vi "Queue MultiPakect-13.vi"(8 "no error":errorcluster, 10 "VISA resource name - IN":refnum<visa-resource-name>="COM4", 11 "EndSession":bool=TRUE) -> (0 "error out":errorcluster={"status"=FALSE, "code"=1073676294, "source"="VISA Read in SerialCOM.vi->Queue MultiPakect-13.vi->getvideo.vi->Focus Routine.vi->Focus Routine.vi.ProxyCaller"}, 1 "success?":bool=TRUE, 2 "ImageData":u8[](array[numeric]) format="%x", 5 "RecvBuff":string, 6 "Done":bool=TRUE, 9 "VISA resource name - OUT":refnum<visa-resource-name>="COM4")   [LabVIEW 2014]
doc: "Demonstrates general use of Obtain Queue, queues and the effects different settings have on queue behavior. It uses a queue to pass data between an Enqueue loop (producing data) and a Dequeue loop (consuming data). If both loops run at the same speed, the queue does not fill up.\n\nWhen the Enqueue loop runs fast and the Dequeue loop runs slow, the queue quickly fills up and the Enqueue loop must wait for the Dequeue loop to remove elements. If the Enqueue loop runs slow and the Dequeue loop runs fast, the queue is quickly emptied and the Dequeue loop must wait for the Enqueue loop to insert elements."
panel:
  out "SendEndSession":bool
  out "max":u32
  out "Raw Data":u8[](array[numeric]) format="%x"
  out "Num_images":dbl=2.0
  out "readtime 2":u32=395
  out "RecvBuff 2":string
  out "ACK 2":bool=TRUE
  out "ACK":bool
  out "#Ends":u32
  out "source":string="VISA Read in SerialCOM.vi->Queue MultiPakect-13.vi->getvideo.vi->Focus Routine.vi->Focus Routine.vi.ProxyCaller"
  out "Pakect":u8[](array[numeric])=[152, 180, 0, 0, 18, 18, 18, 18, 19, 18, 19, 18, 18, 19, 18, 19, 18, 18, 18, 18, 18, 19, 18, 18, 18, 18, 18, 18, 18, 18, 18, 18, 18, 18, 19, 18, 19, 18, 18, 18, 18, 18, 19, 18, 18, 18, 18, 18, 18, 18, 18, 18, 19, 19, 18, 18, 18, 18, 19, 19, 18, 19, 18, 18, 18, 18, 18, 18, 18, 18, 18, 18, 19, 18, 19, 18, 19, 18, 19, 18, 18, 18, 18, 19, 18, 19, 18, 18, 18, 19, 19, 18, 18, 18, 18, 18, 18, 18, 18, 18, 18, 19, 18, 18, 18, 18, 18, 18, 19, 18, 18, 18, 19, 18, 18, 18, 19, 19, 18, 18, 18, 18, 19, 19, 18, 18, 18, 19, 19, 18, 18, 18, 18, 19, 18, 18, 18, 18, 18, 18, 18, 18, 18, 19, 18, 18, 18, 19, 18, 18, 18, 18, 244, 43]
  out "End paks":bool=TRUE
  out "Index":u32=200346
  out "#Pakects":u32=783
  out "# in queue":i32
  out "readtime":u32=395
  out "DeEnque Loop":i32=879
  out "StartTime":u32=22222026
  out "Bytes At Port Loop":i32=1757
  out "Bytes at Port":u32
  out "Enque Loop":i32=391
  out "Bytes Read":u32=200346
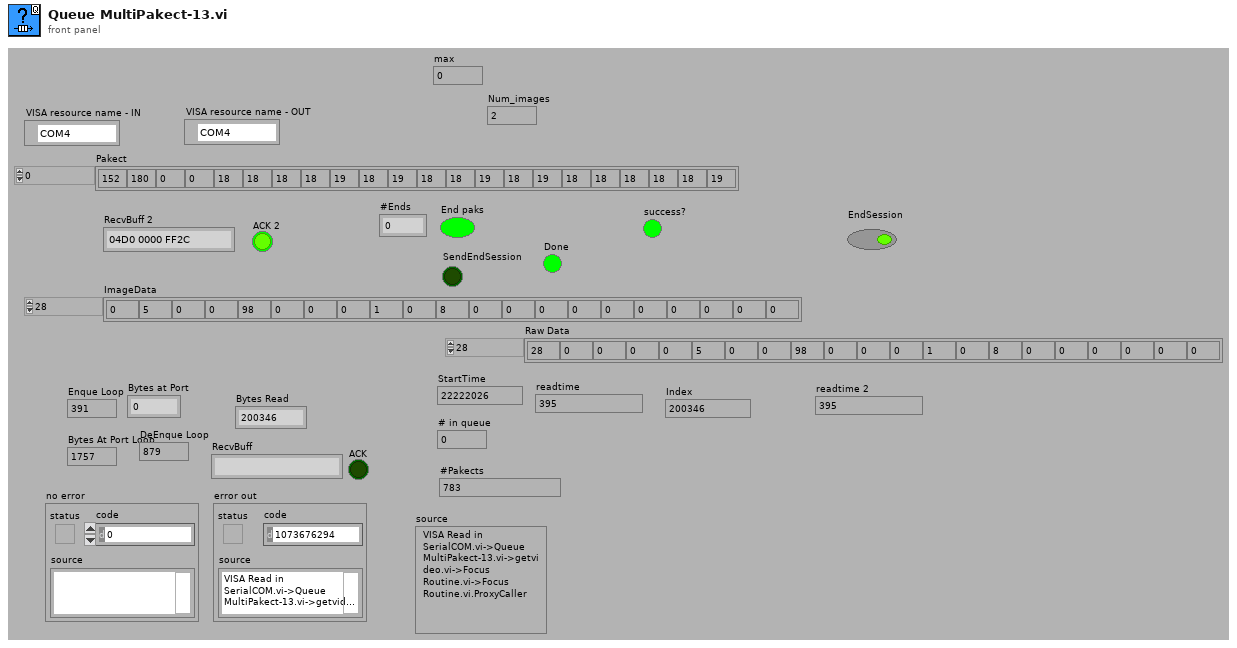
[diagram p1: front panel]
types:
  T1 = enum16{"OpenPort", "Initial Serial Port", "Write", "ByteRead", "Read", "ClearBuff", "Close"}
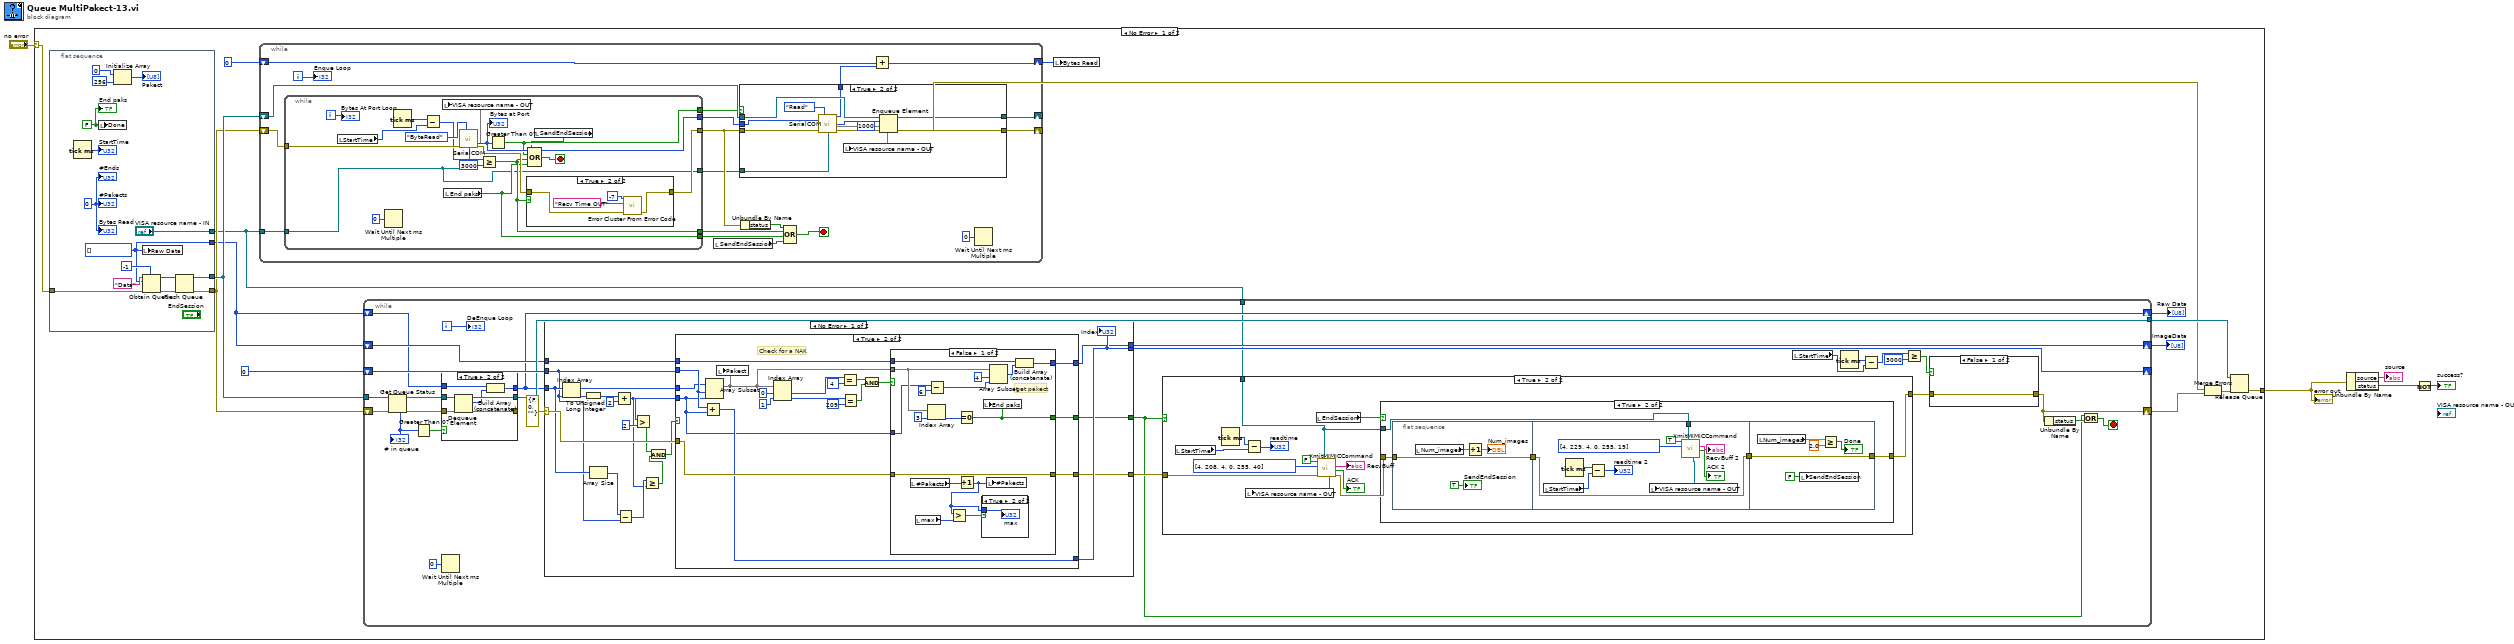
[diagram p0: block diagram]
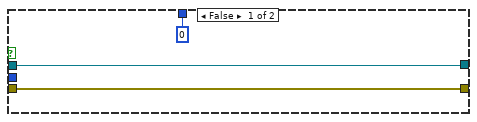
[diagram p3: hidden frame]
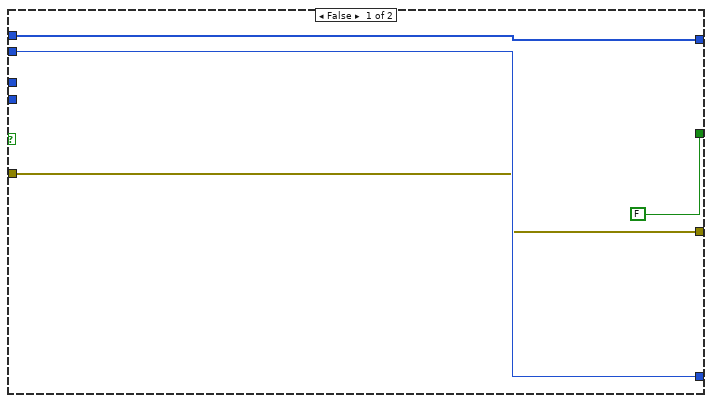
[diagram p4: hidden frame]
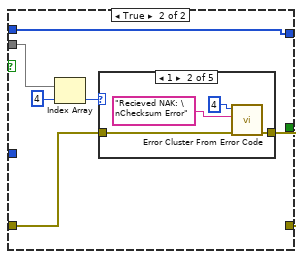
[diagram p6: hidden frame]
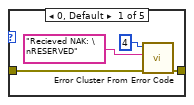
[diagram p7: hidden frame]
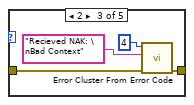
[diagram p8: hidden frame]
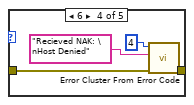
[diagram p9: hidden frame]
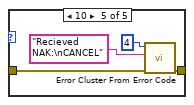
[diagram p10: hidden frame]
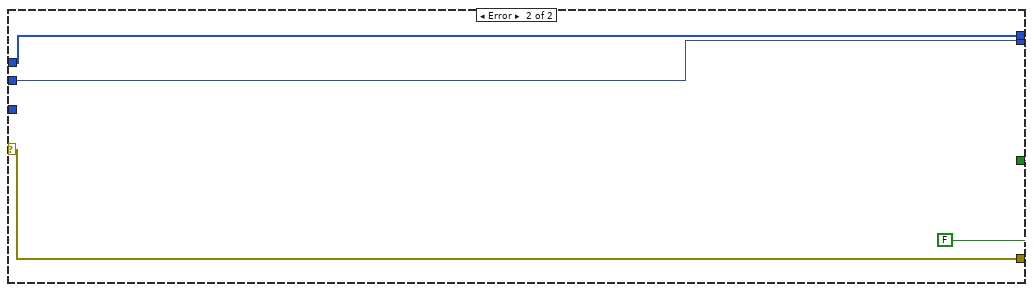
[diagram p11: hidden frame]
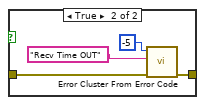
[diagram p12: hidden frame]
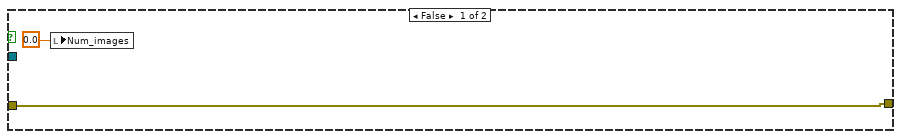
[diagram p15: hidden frame]
diagram:
  n1 = case shown="No Error" "no error" {
    selector: "no error" -> [w11 w264]
    tunnel: [w10 w264] -> w2
    frame No Error {
      n2 = flat-sequence {
        tunnel: [w31] -> w17
        tunnel: [w29] -> w9
        tunnel: [w28] -> w7
        tunnel: w11 -> [w23]
        tunnel: ["VISA resource name - IN"] -> w6
        frame #0 {
          w22 = u32 0 ("Bytes Read")
          w24 = FALSE ("full")
          w28 = u8[] []
          n3 = Tick Count (ms)() -> (millisecond timer value=→"StartTime":u32)
          n4 = local write "Done"(w24) -> ()
          n5 = Initialize Array(u8 0 ("element"), 256 ("dimension size")) -> (→"Pakect":u8[])
          n6 = local write "Raw Data"(w28) -> ()
          n7 = Obtain Queue(max queue size (-1, unlimited)=-1, name (unnamed)="Data", element data type=w28, error in (no error)=w23) -> (queue out=w32:refnum<queue>, error out=w30:errorcluster)  [unwired: 1 in, 1 out]
          n8 = Flush Queue(queue=w32, error in (no error)=w30) -> (queue out=w31:refnum<queue>, error out=w29:errorcluster)  [unwired: 1 out]
          "Bytes Read" <- w22
          "#Pakects" <- w22
          "End paks" <- w24
          "#Ends" <- w22
        }
      }
      n9 = while {
        shift-right: [w51] -> w20
        shift-left: u32 0 ("Bytes Read") -> [w53]
        shift-right: [w49] -> w14
        shift-left: w9 -> [w50]
        shift-right: [w43] -> _
        shift-left: w17 -> [w54]
        tunnel: w6 -> [w39]
        i -> [w47]
        stop <- w48 stop-if-true
        n10 = while {
          tunnel: [w62] -> w45
          tunnel: [w64] -> w52
          tunnel: w50 -> [w71]
          tunnel: [w61] -> w46
          tunnel: [w59] -> w44
          tunnel: [w60] -> w41
          tunnel: w39 -> [w58]
          tunnel: [w58] -> w38
          i -> [w70]
          stop <- w65 stop-if-true
          n11 = local read "StartTime"() -> (w68:u32)
          n12 = Wait Until Next ms Multiple(millisecond multiple=u32 0 ("milliseconds to wait")) -> ()  [unwired: 1 out]
          n13 = Tick Count (ms)() -> (millisecond timer value=w69:u32)
          n14 = Subtract(x=w69, y=w68) -> (x-y=w67:u32)
          n15 = local read "End paks"() -> (w59:bool)
          n16 = call "SerialCOM.vi"("Function"=T1."ByteRead", "error in (no error)"=w71, "VISA_IN"=w58) -> ("Bytes at Port"=w64:u32, 14:w57, "error out"=w63:errorcluster)  [unwired: 6 in, 4 out]
          "Bytes at Port" <- w64
          n17 = local write "VISA resource name - OUT"(w57) -> ()
          n18 = Greater Or Equal?(x=w67, y=u32 3000) -> (x >= y?=w60:bool)
          n19 = Greater Than 0?(x=w64) -> (x > 0?=w61:bool)
          n20 = case shown="True" w60 {
            tunnel: w63 -> [w73 w77]
            tunnel: [w73 w76] -> w62
            frame False {
            }
            frame True {
              n21 = call <vilib>:"Error Cluster From Error Code.vi"("error in (no error)"=w77, "error message (\"\")"="Recv Time OUT" ("error message (\"\")"), "error code (0)"=-7) -> ("error out"=w76:errorcluster)  [unwired: 6 in]
            }
          }
          n22 = local read "SendEndSession"() -> (w55:bool)
          n23 = Compound Arithmetic op=OR(w55, w61, w60, w59) -> (w65:bool)
          "Bytes At Port Loop" <- w70
        }
        n24 = local read "SendEndSession"() -> (w37:bool)
        n25 = case shown="True" w46 {
          tunnel: w45 -> [w80 w89]
          tunnel: w52 -> [_ w87]
          tunnel: w54 -> [w79 w91]
          tunnel: [w80 w85] -> w49
          tunnel: [w79 w86] -> w43
          tunnel: [u32 0 ("return count") w88] -> w42
          tunnel: w38 -> [_ w83]
          frame False {
          }
          frame True {
            n26 = call "SerialCOM.vi"("Function"=T1."Read", "byte count"=w87, "error in (no error)"=w89, "VISA_IN"=w83) -> ("return count"=w88:u32, "array Out"=w84:u8[], 14:w82, "error out"=w90:errorcluster)  [unwired: 5 in, 3 out]
            n27 = local write "VISA resource name - OUT"(w82) -> ()
            n28 = Enqueue Element(queue=w91, element=w84, timeout in ms (-1)=1000, error in (no error)=w90) -> (queue out=w86:refnum<queue>, error out=w85:errorcluster)  [unwired: 1 out]
          }
        }
        n29 = Unbundle By Name(w45) -> ("status"=w40:bool)
        n30 = Compound Arithmetic op=OR(w40, w41, w44, w37) -> (w48:bool)
        n31 = Add(x=w53, y=w42) -> (x+y=w51:u32)
        n32 = Wait Until Next ms Multiple(millisecond multiple=u32 0 ("milliseconds to wait")) -> ()  [unwired: 1 out]
        "Enque Loop" <- w47
      }
      n33 = while {
        tunnel: w17 -> [w119]
        tunnel: [w114] -> w18
        shift-right: [w106] -> w13
        shift-left: w9 -> [w120]
        shift-right: [w113] -> _
        shift-left: u32 0 ("#Pakects") -> [w117]
        shift-right: [w104] -> w12
        shift-left: w7 -> [w105]
        shift-right: [w97] -> w8
        shift-left: w7 -> [w96]
        tunnel: w6 -> [w94]
        i -> [w118]
        stop <- w101 stop-if-true
        n34 = Get Queue Status(queue=w119, error in (no error)=w120) -> (queue out=w115:refnum<queue>, error out=w116:errorcluster, # elements in queue=w98:i32)  [unwired: 1 in, 5 out]
        "# in queue" <- w98
        n35 = Greater Than 0?(x=w98) -> (x > 0?=w99:bool)
        n36 = Wait Until Next ms Multiple(millisecond multiple=u32 0 ("milliseconds to wait")) -> ()  [unwired: 1 out]
        n37 = case shown="True" w99 {
          tunnel: w116 -> [w215 w218]
          tunnel: [w215 w217] -> _
          tunnel: w115 -> [w216 w223]
          tunnel: [w216 w222] -> w114
          tunnel: w96 -> [w214 w221]
          tunnel: [w214 w219] -> w97
          frame False {
          }
          frame True {
            n38 = Dequeue Element(queue=w223, error in (no error)=w218) -> (queue out=w222:refnum<queue>, element=w220:u8[], error out=w217:errorcluster)  [unwired: 2 out]
            n39 = Build Array (concatenate)(w221, w220) -> (w219:u8[])
          }
        }
        n40 = case shown="No Error" errorcluster {"status"=FALSE, "code"=0, "source"=""} ("error IO") {
          selector: errorcluster {"status"=FALSE, "code"=0, "source"=""} ("error IO") -> [w129 w208]
          tunnel: w117 -> [w121 w206]
          tunnel: [w135 w206] -> w113
          tunnel: [w134 w208] -> w112
          tunnel: w105 -> [w132 w207]
          tunnel: [w131 w207] -> w104
          tunnel: w97 -> [w128 _]
          tunnel: [w130 FALSE] -> w102
          frame No Error {
            n41 = Index Array(array=w128, index=w121) -> (element=w136:u8)
            n42 = To Unsigned Long Integer(number=w136) -> (unsigned 32bit integer=w137:u32)
            n43 = Array Size(array=w128) -> (size(s)=w127:i32)
            n44 = Add(x=w137, y=u32 2) -> (x+y=w122:u32)
            n45 = Subtract(x=w127, y=w121) -> (x-y=w123:u32)
            n46 = Greater?(x=w122, y=u32 2) -> (0:w126:bool)
            n47 = Greater Or Equal?(x=w123, y=w122) -> (x >= y?=w125:bool)
            n48 = And(x=w126, y=w125) -> (x .and. y?=w124:bool)
            n49 = case shown="True" w124 {
              tunnel: [w139 w155] -> w131
              tunnel: w121 -> [w141 w153]
              tunnel: w129 -> [w140 w152]
              tunnel: [w141 w148] -> w135
              tunnel: [w140 w147] -> w134
              tunnel: w128 -> [_ w146]
              tunnel: [FALSE w145] -> w130
              tunnel: w122 -> [_ w144]
              tunnel: w132 -> [w139 w143]
              frame False {
              }
              frame True {
                # "Check for a NAK"
                n50 = Add(x=w153, y=w144) -> (x+y=w148:u32)
                n51 = Array Subset(array=w146, index=w153, length=w144) -> (w149:u8[])
                n52 = local write "Pakect"(w149) -> ()
                n53 = Index Array(array=w149, index #1=0 ("index"), index #2=1 ("index")) -> (element #1=w161:u8, element #2=w150:u8)
                n54 = Equal?(x=w161, y=u8 4) -> (x = y?=w157:bool)
                n55 = Equal?(x=w150, y=u8 209) -> (x = y?=w158:bool)
                n56 = Compound Arithmetic op=AND(w157, w158) -> (w154:bool)
                n57 = case shown="False" w154 {
                  tunnel: [w168 w179] -> w155
                  tunnel: w149 -> [w172 w182]
                  tunnel: w144 -> [w171 _]
                  tunnel: w152 -> [w174 w184]
                  tunnel: [w174 w180] -> w147
                  tunnel: [w166 _] -> w145
                  tunnel: w143 -> [w167 w179]
                  frame False {
                    # "get pakect"
                    n58 = local read "#Pakects"() -> (w165:u32)
                    n59 = local read "max"() -> (w162:u32)
                    n60 = Subtract(x=w171, y=u32 6) -> (x-y=w175:u32)
                    n61 = Index Array(array=w172, index=3) -> (element=w170:u8)
                    n62 = Equal To 0?(x=w170) -> (x = 0?=w166:bool)
                    n63 = Increment(x=w165) -> (x+1=w163:u32)
                    n64 = Greater?(x=w163, y=w162) -> (0:w164:bool)
                    n65 = case shown="True" w164 {
                      tunnel: w163 -> [_ w178]
                      frame False {
                      }
                      frame True {
                        "max" <- w178
                      }
                    }
                    n66 = local write "End paks"(w166) -> ()
                    n67 = local write "#Pakects"(w163) -> ()
                    n68 = Array Subset(array=w172, index=4, length=w175) -> (w169:u8[])
                    n69 = Build Array (concatenate)(w167, w169) -> (w168:u8[])
                  }
                  frame True {
                    n70 = Index Array(array=w182, index=4) -> (element=w181:u8)
                    n71 = case shown="1" w181 {
                      tunnel: w184 -> [w188 w192 w196 w200 w204]
                      tunnel: [w187 w191 w195 w199 w203] -> w180
                      frame 0, Default {
                        n72 = call <vilib>:"Error Cluster From Error Code.vi"("error in (no error)"=w188, "error message (\"\")"="Recieved NAK: \nRESERVED" ("error message (\"\")"), "error code (0)"=4) -> ("error out"=w187:errorcluster)  [unwired: 6 in]
                      }
                      frame 1 {
                        n73 = call <vilib>:"Error Cluster From Error Code.vi"("error in (no error)"=w192, "error message (\"\")"="Recieved NAK: \nChecksum Error" ("error message (\"\")"), "error code (0)"=4) -> ("error out"=w191:errorcluster)  [unwired: 6 in]
                      }
                      frame 2 {
                        n74 = call <vilib>:"Error Cluster From Error Code.vi"("error in (no error)"=w196, "error message (\"\")"="Recieved NAK: \nBad Context" ("error message (\"\")"), "error code (0)"=4) -> ("error out"=w195:errorcluster)  [unwired: 6 in]
                      }
                      frame 6 {
                        n75 = call <vilib>:"Error Cluster From Error Code.vi"("error in (no error)"=w200, "error message (\"\")"="Recieved NAK: \nHost Denied" ("error message (\"\")"), "error code (0)"=4) -> ("error out"=w199:errorcluster)  [unwired: 6 in]
                      }
                      frame 10 {
                        n76 = call <vilib>:"Error Cluster From Error Code.vi"("error in (no error)"=w204, "error message (\"\")"="Recieved NAK:\nCANCEL" ("error message (\"\")"), "error code (0)"=4) -> ("error out"=w203:errorcluster)  [unwired: 6 in]
                      }
                    }
                  }
                }
              }
            }
            "Index" <- w135
          }
          frame Error {
          }
        }
        n77 = case shown="True" w102 {
          tunnel: w112 -> [w224 w236]
          tunnel: [w224 w227] -> w100
          tunnel: w94 -> [_ w226]
          frame False {
          }
          frame True {
            n78 = local read "StartTime"() -> (w233:u32)
            n79 = Tick Count (ms)() -> (millisecond timer value=w234:u32)
            n80 = Subtract(x=w234, y=w233) -> (x-y=→"readtime":u32)
            n81 = local read "EndSession"() -> (w228:bool)
            n82 = call "XmitMIMICCommand.vi"("VISA resource name - IN"=w226, "error in (no error)"=w236, "Command array"=u8[] [4, 208, 4, 0, 255, 40], "ACK?"=FALSE) -> ("error out"=w229:errorcluster, "ACK"=→"ACK":bool, "RecvBuff"=→"RecvBuff":string, "VISA resource name - OUT"=w225:refnum<visa-resource-name>)  [unwired: 1 in, 1 out]
            n83 = local write "VISA resource name - OUT"(w225) -> ()
            n84 = case shown="True" w228 {
              tunnel: w229 -> [w239 w243]
              tunnel: [w239 w241] -> w227
              tunnel: w226 -> [_ w240]
              frame False {
                n85 = local write "Num_images"(0.0 ("Num_images")) -> ()
              }
              frame True {
                n86 = flat-sequence {
                  tunnel: [w246] -> w244
                  tunnel: w243 -> [w246]
                  tunnel: w244 -> [w251]
                  tunnel: [w251] -> w242
                  tunnel: w240 -> [w250]
                  tunnel: w242 -> [w260]
                  tunnel: [w260] -> w241
                  frame #0 {
                    n87 = local read "Num_images"() -> (w247:dbl)
                    n88 = Increment(x=w247) -> (x+1=→"Num_images":dbl)
                    "SendEndSession" <- TRUE ("SendEndSession")
                  }
                  frame #1 {
                    n89 = local read "StartTime"() -> (w255:u32)
                    n90 = Tick Count (ms)() -> (millisecond timer value=w254:u32)
                    n91 = Subtract(x=w254, y=w255) -> (x-y=→"readtime 2":u32)
                    n92 = call "XmitMIMICCommand.vi"("VISA resource name - IN"=w250, "Command array"=u8[] [4, 229, 4, 0, 255, 19], "ACK?"=TRUE) -> ("ACK"=→"ACK 2":bool, "RecvBuff"=→"RecvBuff 2":string, "VISA resource name - OUT"=w249:refnum<visa-resource-name>)  [unwired: 2 in, 2 out]
                    n93 = local write "VISA resource name - OUT"(w249) -> ()
                  }
                  frame #2 {
                    n94 = local read "Num_images"() -> (w261:dbl)
                    n95 = local write "SendEndSession"(FALSE ("SendEndSession")) -> ()
                    n96 = Greater Or Equal?(x=w261, y=2.0) -> (x >= y?=→"Done":bool)
                  }
                }
              }
            }
          }
        }
        n97 = local read "StartTime"() -> (w108:u32)
        n98 = Tick Count (ms)() -> (millisecond timer value=w109:u32)
        n99 = Subtract(x=w109, y=w108) -> (x-y=w110:u32)
        n100 = Greater Or Equal?(x=w110, y=u32 3000) -> (x >= y?=w107:bool)
        n101 = case shown="False" w107 {
          tunnel: w100 -> [w209 w213]
          tunnel: [w209 w212] -> w106
          frame False {
          }
          frame True {
            n102 = call <vilib>:"Error Cluster From Error Code.vi"("error in (no error)"=w213, "error message (\"\")"="Recv Time OUT" ("error message (\"\")"), "error code (0)"=-5) -> ("error out"=w212:errorcluster)  [unwired: 6 in]
          }
        }
        n103 = Unbundle By Name(w106) -> ("status"=w103:bool)
        n104 = Compound Arithmetic op=OR(w102, w103) -> (w101:bool)
        "DeEnque Loop" <- w118
      }
      "ImageData" <- w12
      "Raw Data" <- w8
      n105 = local write "Bytes Read"(w20) -> ()
      n106 = Merge Errors(w14, w13) -> (w19:errorcluster)
      n107 = Release Queue(queue=w18, error in (no error)=w19) -> (error out=w10:errorcluster)  [unwired: 3 out]
    }
    frame Error {
    }
  }
  "error out" <- w2
  n108 = Unbundle By Name(w2) -> ("source"=→"source":string, "status"=w4:bool)
  n109 = Not(x=w4) -> (.not. x?=→"success?":bool)
